vi "SetVelSingleAxis.vi"(1 "Vel":dbl format="%.2f", 2 "Axis":i32=1) -> (0 "Command executed":bool)   [LabVIEW 2015, in "DLLS4.lvclass"]
uses:
  Classes/Delay Line/DelayLineLS4/DLLS4.lvclass
  DLL/LStep4.dll
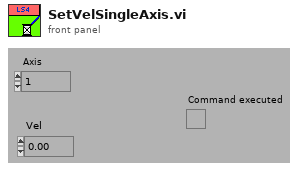
[diagram p1: front panel]
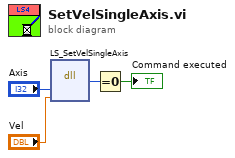
[diagram p0: block diagram]
diagram:
  n1 = dll-call lib="C:/Users/Sergey Denisov/Documents/REPS/TRANCON/DLL/LStep4.dll" fn="LS_SetVelSingleAxis"("Axis"="Axis", "Vel"="Vel") -> ("type de retour"=w3:i32)  [unwired: 5 in, 2 out]
  n2 = Equal To 0?(x=w3) -> (x = 0?=→"Command executed":bool)
